vi "linearfit.vi"(9 "index 2":i32, 10 "index":i32, 11 "array":dbl[](array[numeric])) -> (1 "intercept":dbl, 3 "slope":dbl)   [LabVIEW 2015]
uses:
  <vilib>/Analysis/baseanly.llb/Mean (DBL).vi
  <vilib>/Analysis/NI_AALBase.lvlib
  <vilib>/Analysis/NI_AALPro.lvlib
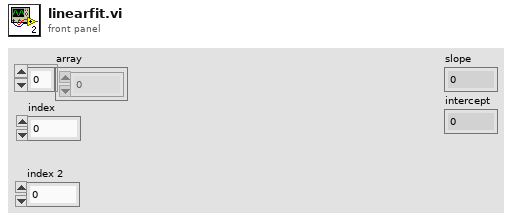
[diagram p1: front panel]
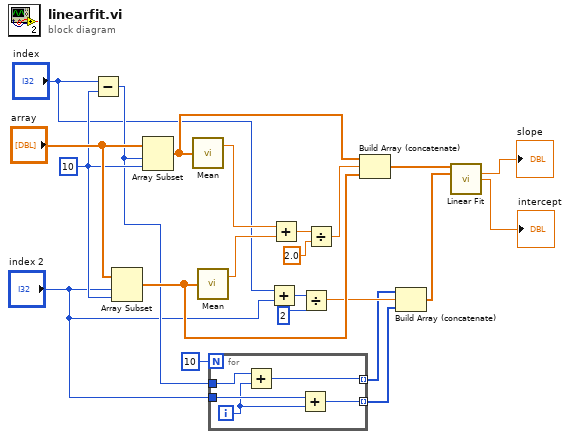
[diagram p0: block diagram]
diagram:
  w21 = 10 ("length")
  n1 = Subtract(x="index", y=w21) -> (x-y=w11:i32)
  n2 = Array Subset(array="array", index="index 2", length=w21) -> (w14:dbl[])
  n3 = Array Subset(array="array", index=w11, length=w21) -> (w16:dbl[])
  n4 = call-poly <vilib>:"Mean.vi"("X"=w16) -> ("mean"=w20:dbl)  [unwired: 1 out]
  n5 = call-poly <vilib>:"Mean.vi"("X"=w14) -> ("mean"=w19:dbl)  [unwired: 1 out]
  n6 = for {
    N: 10 -> [_]
    tunnel: [w26] -> w3 mode=indexing
    tunnel: w11 -> [w27]
    tunnel: "index 2" -> [w25]
    tunnel: [w23] -> w2 mode=indexing
    i -> [w24]
    n7 = Add(x=w27, y=w24) -> (x+y=w26:i32)
    n8 = Add(x=w25, y=w24) -> (x+y=w23:i32)
  }
  n9 = Add(x="index", y="index 2") -> (x+y=w6:i32)
  n10 = Add(x=w20, y=w19) -> (x+y=w18:dbl)
  n11 = Divide(x=w6, y=2) -> (x/y=w4:dbl)
  n12 = Divide(x=w18, y=2.0) -> (x/y=w15:dbl)
  n13 = Build Array (concatenate)(w16, w15, w14) -> (w13:dbl[])
  n14 = Build Array (concatenate)(w3, w4, w2) -> (w1:dbl[])
  n15 = call <vilib>:"Linear Fit.vi"("Y"=w13, "X"=w1) -> ("slope"=→"slope":dbl, "intercept"=→"intercept":dbl)  [unwired: 9 in, 3 out]
